vi "SLL DE File and folder info.vi"(8 "error in (no error)":errorcluster) -> (0 "error out":errorcluster, 1 "Seq File Folder":path, 2 "DAQ INI file path":path, 3 "Report path":path, 5 "Virtual Chart":path, 7 "View File":path)   [LabVIEW 2013]
doc: "Copyright © 2005, Soliton Technologies.\nAll rights reserved."
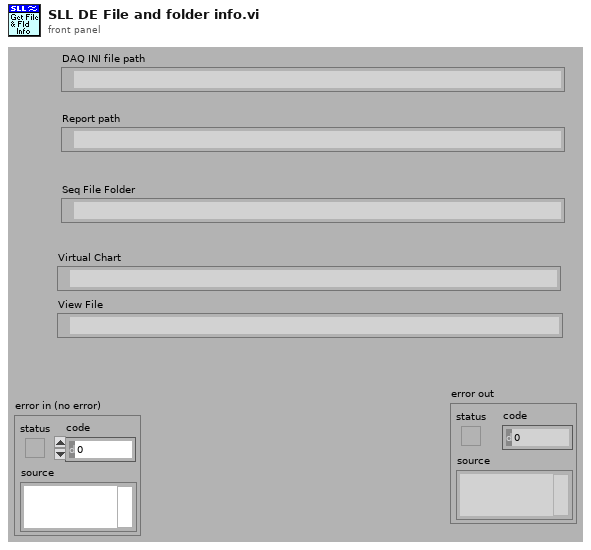
[diagram p1: front panel]
types:
  T1 = enum32{"invalid app kind", "Development System", "Run Time System", "Student Edition", "Embedded LabVIEW", "Evaluation", "Custom"}
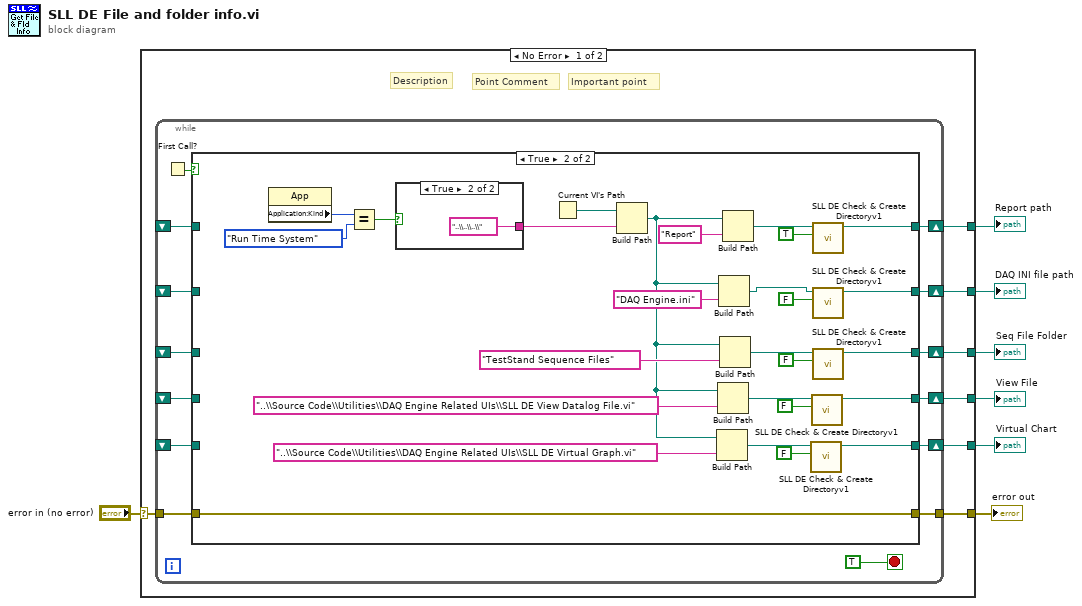
[diagram p0: block diagram]
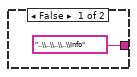
[diagram p3: hidden frame]
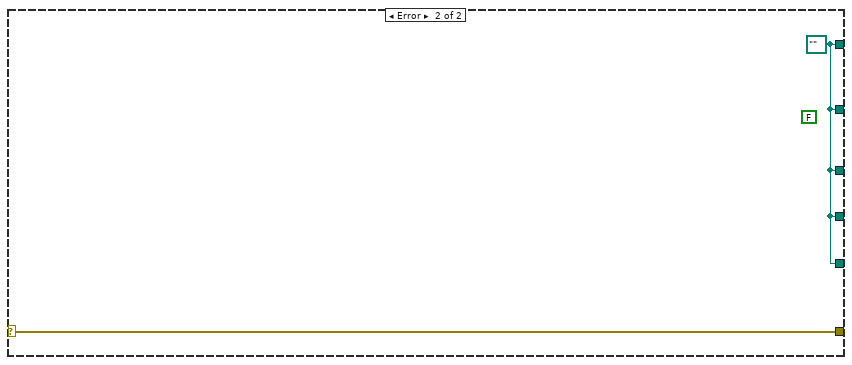
[diagram p4: hidden frame]
diagram:
  n1 = case shown="No Error" "error in (no error)" {
    selector: "error in (no error)" -> [w14 w65]
    tunnel: [w13 w65] -> w6
    tunnel: [w12 w64] -> w5
    tunnel: [w11 w64] -> w4
    tunnel: [w10 w64] -> w3
    tunnel: [w9 w64] -> w2
    tunnel: [w8 w64] -> w1
    frame No Error {
      # "Point Comment"
      # "Important point"
      # "Description"
      n2 = while {
        tunnel: w14 -> [w26]
        tunnel: [w25] -> w13
        shift-right: [w24] -> w12
        shift-left: _ -> [w23]
        shift-right: [w22] -> w11
        shift-left: _ -> [w21]
        shift-right: [w20] -> w10
        shift-left: _ -> [w19]
        shift-right: [w18] -> w9
        shift-left: _ -> [w16]
        shift-right: [w17] -> w8
        shift-left: _ -> [w15]
        stop <- TRUE stop-if-true
        n3 = First Call?() -> (First Call?: T/F=w27:bool)
        n4 = case shown="True" w27 {
          tunnel: w26 -> [w34 w56]
          tunnel: [w34 w56] -> w25
          tunnel: [w33 w52] -> w24
          tunnel: w23 -> [w33 _]
          tunnel: [w32 w50] -> w22
          tunnel: w21 -> [w32 _]
          tunnel: [w31 w44] -> w20
          tunnel: w19 -> [w31 _]
          tunnel: [w30 w36] -> w18
          tunnel: [w29 w35] -> w17
          tunnel: w16 -> [w30 _]
          tunnel: w15 -> [w29 _]
          frame False {
          }
          frame True {
            n5 = property class="App"() -> ("Application:Kind"=w58:T1)  [unwired: 2 in, 2 out]
            n6 = Equal?(x=w58, y=T1."Run Time System") -> (x = y?=w55:bool)
            n7 = case shown="True" w55 {
              tunnel: ["..\\..\\..\\..\\Info" ("name or relative path") "..\\..\\..\\" ("name or relative path")] -> w59
              frame False {
              }
              frame True {
              }
            }
            n8 = Current VI's Path() -> (path=w61:path)
            n9 = Build Path(base path=w61, name or relative path=w59) -> (appended path=w38:path)
            n10 = Build Path(base path=w38, name or relative path="..\\Source Code\\Utilities\\DAQ Engine Related UIs\\SLL DE Virtual Graph.vi") -> (appended path=w39:path)
            n11 = Build Path(base path=w38, name or relative path="..\\Source Code\\Utilities\\DAQ Engine Related UIs\\SLL DE View Datalog File.vi") -> (appended path=w43:path)
            n12 = Build Path(base path=w38, name or relative path="DAQ Engine.ini") -> (appended path=w48:path)
            n13 = Build Path(base path=w38, name or relative path="TestStand Sequence Files") -> (appended path=w46:path)
            n14 = Build Path(base path=w38, name or relative path="Report") -> (appended path=w53:path)
            n15 = call "SLL DE Check & Create Directoryv1.vi"("Path is Directory? (F=No)"=FALSE, "Path"=w39) -> ("Dup Path out"=w35:path)  [unwired: 8 in, 1 out]
            n16 = call "SLL DE Check & Create Directoryv1.vi"("Path is Directory? (F=No)"=FALSE, "Path"=w43) -> ("Dup Path out"=w36:path)  [unwired: 8 in, 1 out]
            n17 = call "SLL DE Check & Create Directoryv1.vi"("Path is Directory? (F=No)"=TRUE, "Path"=w53) -> ("Dup Path out"=w52:path)  [unwired: 8 in, 1 out]
            n18 = call "SLL DE Check & Create Directoryv1.vi"("Path is Directory? (F=No)"=FALSE, "Path"=w48) -> ("Dup Path out"=w50:path)  [unwired: 8 in, 1 out]
            n19 = call "SLL DE Check & Create Directoryv1.vi"("Path is Directory? (F=No)"=FALSE, "Path"=w46) -> ("Dup Path out"=w44:path)  [unwired: 8 in, 1 out]
          }
        }
      }
    }
    frame Error {
      w64 = path "" ("appended path")
      (unwired) FALSE ("Newly created?")
    }
  }
  "error out" <- w6
  "Report path" <- w5
  "DAQ INI file path" <- w4
  "Seq File Folder" <- w3
  "View File" <- w2
  "Virtual Chart" <- w1
